vi "Write Sub panel msg.vi"(8 "error in (no error)":errorcluster, 10 "Sub panel msg":refnum<vi>, 11 "Mensaje Actor in":refnum<class "Mensaje Actor.lvclass">) -> (0 "error out":errorcluster, 3 "Mensaje Actor out":refnum<class "Mensaje Actor.lvclass">)   [LabVIEW 2019, in "Mensaje Actor.lvlib" / "Mensaje Actor.lvclass"]
uses:
  Mensaje Actor.lvclass
  Mensaje Actor.lvclass/Mensaje Actor.ctl
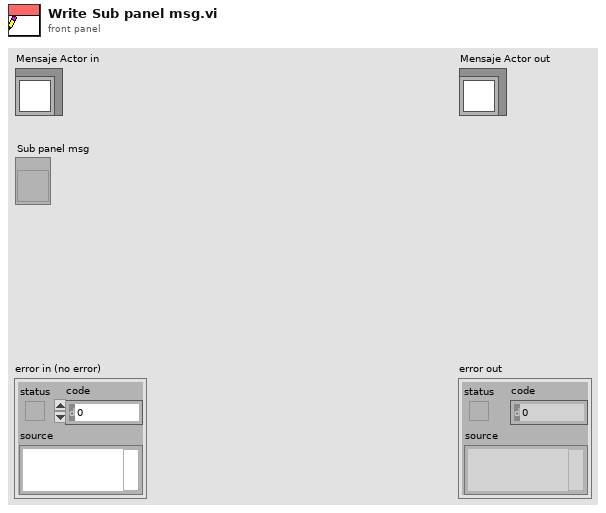
[diagram p1: front panel]
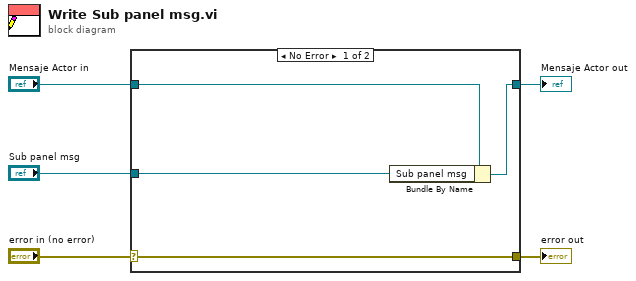
[diagram p0: block diagram]
diagram:
  n1 = case shown="No Error" "error in (no error)" {
    selector: "error in (no error)" -> [w9 w10]
    tunnel: [w9 w10] -> w4
    tunnel: [w7 w11] -> w2
    tunnel: "Mensaje Actor in" -> [w8 w11]
    tunnel: "Sub panel msg" -> [w6 _]
    frame No Error {
      n2 = Bundle By Name(cluster=w8, "Sub panel msg"=w6) -> (w7:refnum<class "Mensaje Actor.lvclass">)
    }
    frame Error {
    }
  }
  "error out" <- w4
  "Mensaje Actor out" <- w2
